vi "PI.vi"(0 "Threshold":dbl=0.5, 2 "Current at Steady State":dbl=5.5, 4 "Tasking Period":dbl, 5 "Kp":dbl, 6 "Reference Speed (rad/s)":dbl, 7 "Ki":dbl, 8 "Real Speed (rad/s)":dbl, 9 "No Kf":bool, 10 "Kf":dbl min=0.0, 11 "Error In":errorcluster) -> (1 "PI Current (A)":dbl, 3 "Error Out":errorcluster)   [LabVIEW 2021]
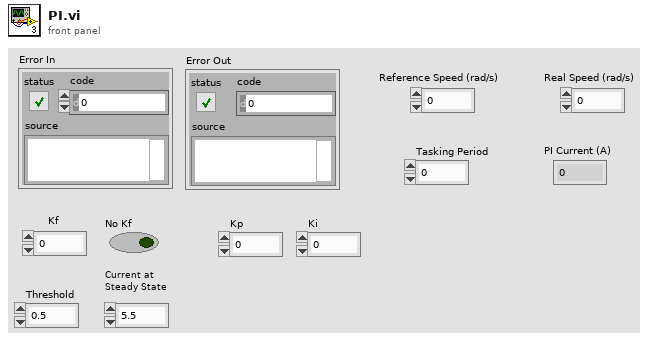
[diagram p1: front panel]
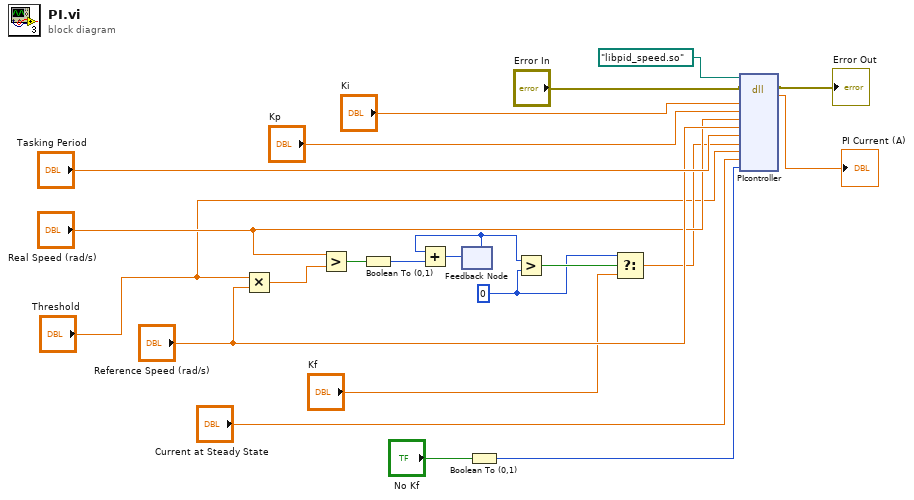
[diagram p0: block diagram]
diagram:
  w7 = 0
  n1 = Multiply(x="Threshold", y="Reference Speed (rad/s)") -> (x*y=w13:dbl)
  n2 = Greater?(x="Real Speed (rad/s)", y=w13) -> (0:w12:bool)
  n3 = Boolean To (0,1)(Boolean=w12) -> (0, 1=w11:i16)
  n4 = feedback #1() -> (w9:i16)  [unwired: 1 in]
  n5 = Add(x=w9, y=w11) -> (x+y=w10:i16)
  n6 = feedback-in #1(w10) -> ()
  n7 = Boolean To (0,1)(Boolean="No Kf") -> (0, 1=w3:i16)
  n8 = Greater?(x=w9, y=w7) -> (0:w8:bool)
  n9 = Select(t=w7, s=w8, f="Kf") -> (s? t:f=w4:dbl)
  n10 = dll-call lib="?" fn="PIcontroller"(path in=path "libpid_speed.so", error in="Error In", "Ki"="Ki", "Kp"="Kp", "measured_speed"="Real Speed (rad/s)", "reference_speed"="Reference Speed (rad/s)", "Tasking_period"="Tasking Period", "Kf"=w4, "threshold"="Threshold", "steady_curr"="Current at Steady State", "no_Kf"=w3) -> (error out=→"Error Out":errorcluster, "output"=→"PI Current (A)":sgl)  [unwired: 10 in, 1 out]
